vi "Two niScope EX Getting Started.vi"() -> ()   [LabVIEW 2021]
doc: "Example: Getting Started\n\nRecommended Input Signal: 100 kHz, 1.8 Vpp, sine wave\n\nDevices Supported: Refer to NI Example Finder\n\nLabVIEW Description:\n\nThis example opens a session to the NI-SCOPE driver by passing in the device's resource name to the Initialize VI. The resource name is a unique identifier for your National Instruments' hardware product. It can be found (and changed) by running Measurement & Automation Explorer (MAX). A shortcut to MAX is placed on your desktop when NI-SCOPE or NI-DAQ is installed.\n\nThe session handle returned from the Initialize VI is a parameter to all VIs in the NI-SCOPE driver. Only one session may be opened at a time for your oscilloscope, and every session should be closed by calling the Close vi. The session should be closed even when an error occurs.\n\nThe Auto Setup VI takes several acquisitions to measure the amplitude and frequency of the input signal. This allows it to optimally set properties such as the sample rate, vertical range, and minimum record length. The Read VI, initiates an acquisition, waits for it to finish, and fetches the data from the oscilloscope. The data is returned as a bundle of the initial x, x increment, and waveform. Initial x is the time of the first point in the waveform relative to the trigger, while the x increment is the time between two points in the waveform. This bundle may be directly wired to a waveform graph, to display the waveform with timing information. \n\nThe Error Handler VI translates any error messages into text messages."
uses:
  <instrlib>/niScope/Acquire/niScope Multi Read Cluster.vi
panel:
  in  "error in":errorcluster
  out "error out":errorcluster
  in  "SMU Scope Channel(s)":string="0"
  in  "SMU Scope":refnum<k15>="Dev1"
  out "SMU Scope Waveform Graph":T1(graph)
  out "Load Scope Waveform Graph":T1(graph)
  in  "Load Scope":refnum<k15>="Dev1"
  in  "Load Scope Channel(s)":string="0"
  # "Overview: Demonstrates the minimal code needed to use NI-SCOPE.\nRequirements: NI-SCOPE\nInstructions: \n1.  Select the appropriate device in the Resource Name control.\n2.  Enter the channels you would like to acquire from in the Channel(s) control.\n3.  Run the VI."
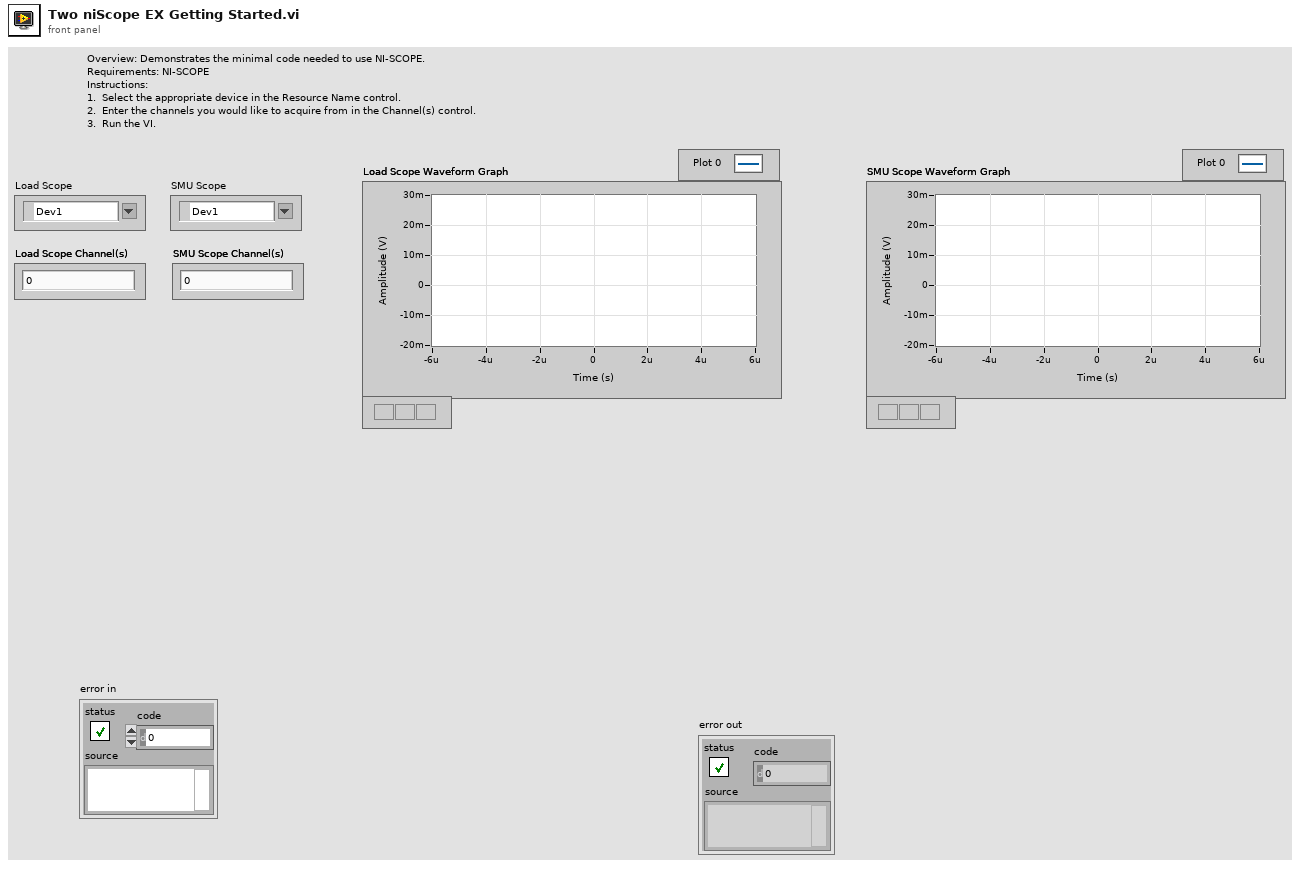
[diagram p1: front panel]
types:
  T1 = cluster{"relativeInitialX":dbl, "xIncrement":dbl, "wfm":dbl[]}[]
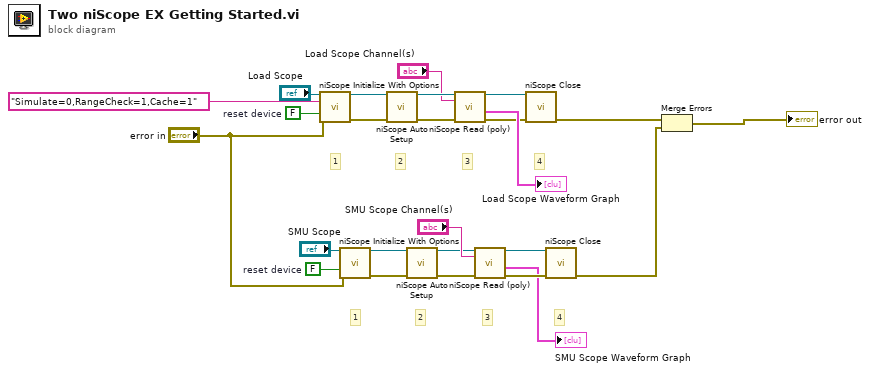
[diagram p0: block diagram]
diagram:
  w8 = FALSE  # reset device
  w22 = FALSE  # reset device
  # "4"
  # "3"
  # "2"
  # "1"
  # "4"
  # "3"
  # "2"
  # "1"
  n1 = call <instrlib>:"niScope Initialize With Options.vi"("resource name"="Load Scope", "option string"="Simulate=0,RangeCheck=1,Cache=1", "reset device"=w22, "error in"="error in") -> ("instrument handle"=w25:refnum<k15>, "error out"=w24:errorcluster)  [unwired: 10 in]
  n2 = call <instrlib>:"niScope Initialize With Options.vi"("resource name"="SMU Scope", "reset device"=w8, "error in"="error in") -> ("instrument handle"=w5:refnum<k15>, "error out"=w6:errorcluster)  [unwired: 11 in]
  n3 = call <instrlib>:"niScope Auto Setup.vi"("instrument handle"=w25, "error in"=w24) -> ("instrument handle out"=w21:refnum<k15>, "error out"=w20:errorcluster)  [unwired: 12 in]
  n4 = call <instrlib>:"niScope Auto Setup.vi"("instrument handle"=w5, "error in"=w6) -> ("instrument handle out"=w9:refnum<k15>, "error out"=w10:errorcluster)  [unwired: 12 in]
  n5 = call-poly <instrlib>:"niScope Read (poly).vi"("error in"=w20, "channels"="Load Scope Channel(s)", "instrument handle"=w21) -> ("error out"=w17:errorcluster, "waveform"=→"Load Scope Waveform Graph":T1, "instrument handle out"=w16:refnum<k15>)  [unwired: 5 in, 1 out]
  n6 = call-poly <instrlib>:"niScope Read (poly).vi"("error in"=w10, "channels"="SMU Scope Channel(s)", "instrument handle"=w9) -> ("error out"=w13:errorcluster, "waveform"=→"SMU Scope Waveform Graph":T1, "instrument handle out"=w14:refnum<k15>)  [unwired: 5 in, 1 out]
  n7 = call <instrlib>:"niScope Close.vi"("instrument handle"=w16, "error in"=w17) -> ("error out"=w4:errorcluster)  [unwired: 13 in]
  n8 = call <instrlib>:"niScope Close.vi"("instrument handle"=w14, "error in"=w13) -> ("error out"=w2:errorcluster)  [unwired: 13 in]
  n9 = Merge Errors(w4, w2) -> (→"error out":errorcluster)
